vi "Plot IPI.vi"(0 "Y":dbl[](array[numeric]), 1 "XYGraph":refnum<vi>) -> ()   [LabVIEW 2020]
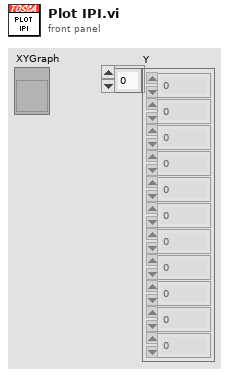
[diagram p1: front panel]
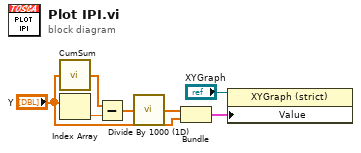
[diagram p0: block diagram]
diagram:
  n1 = call "CumSum.vi"("Array"="Y") -> ("CumSum"=w4:dbl[])
  n2 = Index Array(array="Y") -> (element=w2:dbl)  [unwired: 1 in]
  n3 = Subtract(x=w4, y=w2) -> (x-y=w1:dbl[])
  n4 = call "Divide By 1000 (1D).vi"("X"=w1) -> ("X/1000"=w6:dbl[])
  n5 = Bundle("X/1000"=w6, "Y"="Y") -> (w5:cluster{"X/1000":dbl[], "Y":dbl[]})  [unwired: 1 in]
  n6 = property class="XYGraph (strict)"(reference="XYGraph", "Value"=w5) -> ()  [unwired: 1 in, 2 out]
